vi "Start Sync.vi"(8 "error in (no error)":errorcluster, 11 "gRPC Server in":refnum<class "PluginLoader.lvclass">) -> (0 "error out":errorcluster, 3 "gRPC Server out":refnum<class "PluginLoader.lvclass">)   [LabVIEW 2021, in "CIF_PluginLoader_server.lvlib" / "PluginLoader.lvclass"]
uses:
  PluginLoader.lvclass
  PluginLoader.lvclass/PluginLoader.ctl
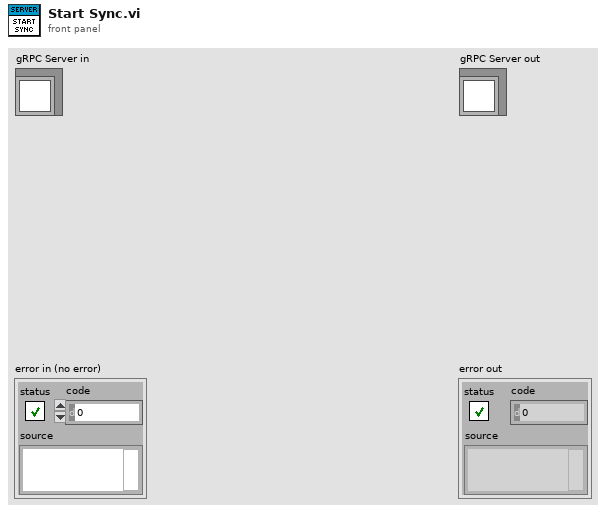
[diagram p1: front panel]
types:
  T1 = typedef "CIF_PluginLoader_server.lvlib/PluginLoader.lvclass/Server Internal UEs.ctl" = cluster{"PluginLoader LoadPlugin Internal UE":refnum<user-event>, "PluginLoader AbortPlugin Internal UE":refnum<user-event>, "PluginLoader Destroy Internal UE":refnum<user-event>, "PluginLoader Ping Internal UE":refnum<user-event>, "PluginLoader Discover Internal UE":refnum<user-event>}
  T2 = typedef "CIF_PluginLoader_server.lvlib/PluginLoader.lvclass/Server gRPC UEs.ctl" = cluster{"PluginLoader LoadPlugin gRPC UE":refnum<user-event>, "PluginLoader AbortPlugin gRPC UE":refnum<user-event>, "PluginLoader Destroy gRPC UE":refnum<user-event>, "PluginLoader Ping gRPC UE":refnum<user-event>, "PluginLoader Discover gRPC UE":refnum<user-event>}
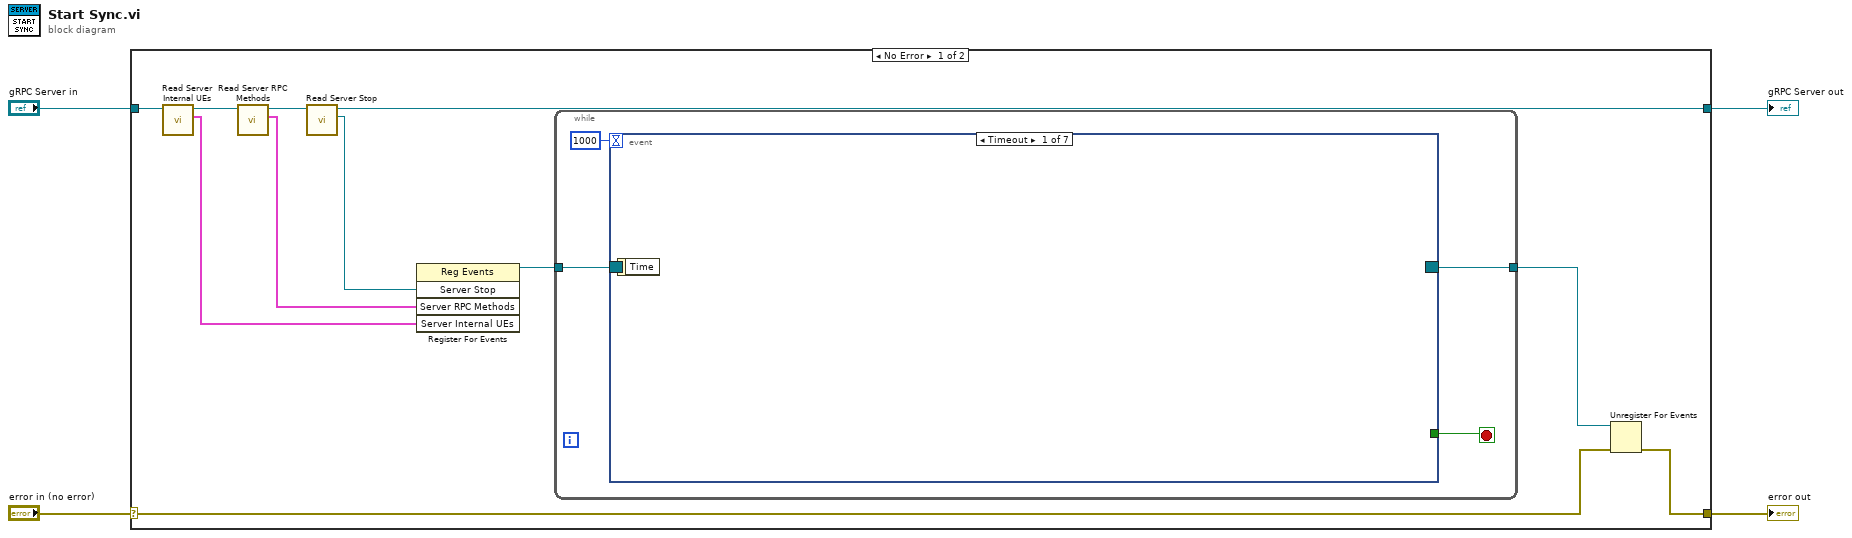
[diagram p0: block diagram]
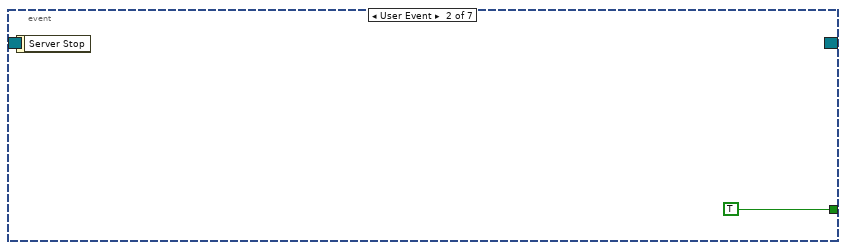
[diagram p2: hidden frame]
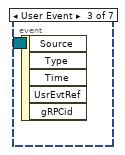
[diagram p3: hidden frame]
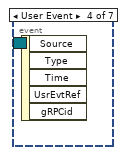
[diagram p4: hidden frame]
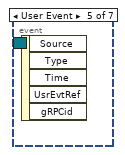
[diagram p5: hidden frame]
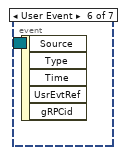
[diagram p6: hidden frame]
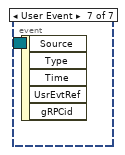
[diagram p7: hidden frame]
diagram:
  n1 = case shown="No Error" "error in (no error)" {
    selector: "error in (no error)" -> [w9 w22]
    tunnel: [w8 w22] -> w3
    tunnel: [w6 w21] -> w1
    tunnel: "gRPC Server in" -> [w15 w21]
    frame No Error {
      n2 = call "Read Server Internal UEs.vi"("SignalGeneratorService in"=w15) -> ("Server Internal UEs"=w13:T1, "SignalGeneratorService out"=w14:refnum<class "PluginLoader.lvclass">)  [unwired: 8 in, 1 out]
      n3 = call "Read Server RPC Methods.vi"("SignalGeneratorService in"=w14) -> ("Server RPC Methods"=w7:T2, "SignalGeneratorService out"=w12:refnum<class "PluginLoader.lvclass">)  [unwired: 8 in, 1 out]
      n4 = call-dynamic "Read Server Stop.vi"("iService in"=w12) -> ("Server Stop"=w5:refnum<user-event>, "iService out"=w6:refnum<class "PluginLoader.lvclass">)  [unwired: 8 in, 1 out]
      n5 = register-events(w5, w7, w13) -> (reference out=w11:refnum<event-registration>)  [unwired: 2 in, 1 out]
      n6 = while {
        tunnel: w11 -> [w19]
        tunnel: [w17] -> w10
        stop <- w18 stop-if-true
        n7 = event "RPC Methods Event Structure" shown="[0] Timeout" {
          selector: w19 -> [_ _ _ _ _ _ _]
          dyn-events: [_ _ _ _ _ _ _] -> w17
          timeout: 1000 -> [_ _ _ _ _ _ _]
          tunnel: [_ TRUE _ _ _ _ _] -> w18
          event Timeout {
            n8 = event-data() -> ()  [unwired: 1 in, 1 out]
          }
          event User Event {
            n9 = event-data() -> ()  [unwired: 1 in, 1 out]
          }
          event User Event {
            n10 = event-data() -> ()  [unwired: 1 in, 5 out]
          }
          event User Event {
            n11 = event-data() -> ()  [unwired: 1 in, 5 out]
          }
          event User Event {
            n12 = event-data() -> ()  [unwired: 1 in, 5 out]
          }
          event User Event {
            n13 = event-data() -> ()  [unwired: 1 in, 5 out]
          }
          event User Event {
            n14 = event-data() -> ()  [unwired: 1 in, 5 out]
          }
        }
      }
      n15 = Unregister For Events(event registration refnum=w10, error in=w9) -> (error out=w8:errorcluster)
    }
    frame Error {
    }
  }
  "error out" <- w3
  "gRPC Server out" <- w1
